vi "Shooter Speed Global.vi"() -> ()   [LabVIEW 2013]
panel:
  in  "Motor Output":dbl
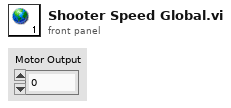
[diagram p1: front panel]
diagram:
